vi "Pointer.Read.vi"   [LabVIEW 2016, in "VeriStand Data.lvlib"]
doc: "Reads a number of values, specified by <B>count</B>, from the provided <B>pointer</B>."
uses:
  VeriStand Data.lvlib
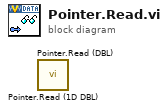
[diagram p0: block diagram]
diagram:
  n1 = call "Pointer.Read (1D DBL).vi"() -> ()  [unwired: 9 in, 3 out]
  n2 = call "Pointer.Read (DBL).vi"() -> ()  [unwired: 9 in, 3 out]
